vi "test_rw_string.vi"(8 "error in (no error)":errorcluster) -> (0 "error out":errorcluster)   [LabVIEW 2020]
uses:
  75441b51-3bf2-4981-8bbc-1672bc4a7a0b.vi
  75441b51-3bf2-4981-8bbc-1672bc4a7a0b.vi/4178f046-9af6-4db4-9405-99552d650b27.vi
  75441b51-3bf2-4981-8bbc-1672bc4a7a0b.vi/504846f3-46c1-483c-ab2c-e4b1da560c38.vi
  toml/write_subtable_key_string.vi
  toml/toml.lvclass
  <vilib>/addons/_JKI Toolkits/Caraya/classes/Assert/Assert.lvclass
  <vilib>/addons/_JKI Toolkits/Caraya/classes/Test/Test.lvclass
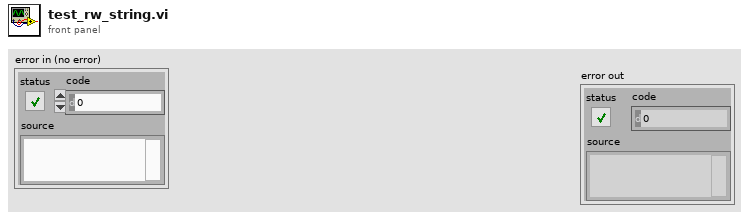
[diagram p1: front panel]
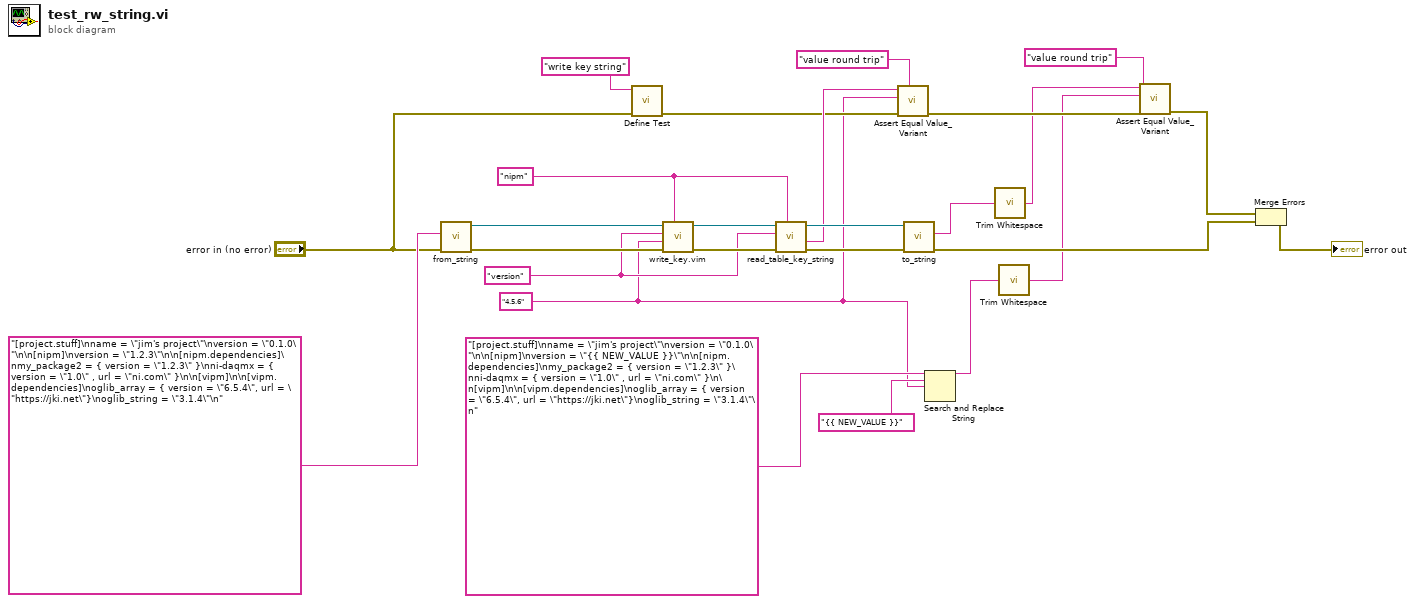
[diagram p0: block diagram]
diagram:
  w2 = "version" ("table_name")
  w3 = "nipm" ("table_name")
  w1 = "4.5.6" ("string")
  n1 = call "from_string.vi"("error in (no error)"="error in (no error)", "toml"="[project.stuff]\nname = \"jim's project\"\nversion = \"0.1.0\"\n\n[nipm]\nversion = \"1.2.3\"\n\n[nipm.dependencies]\nmy_package2 = { version = \"1.2.3\" }\nni-daqmx = { version = \"1.0\" , url = \"ni.com\" }\n\n[vipm]\n\n[vipm.dependencies]\noglib_array = { version = \"6.5.4\", url = \"https://jki.net\"}\noglib_string = \"3.1.4\"\n" ("toml_string in")) -> ("error out"=w21:errorcluster, "toml out"=w20:refnum<class "toml.lvclass">)  [unwired: 8 in]
  n2 = call <vilib>:"Define Test.vi"("error in (no error)"="error in (no error)", "Label (VI Title)"="write key string") -> ("error out"=w9:errorcluster)  [unwired: 9 in]
  n3 = call "write_key.vim"("table"=w3, "error in (no error)"=w21, "value"=w1, "key"=w2, "toml in"=w20) -> ("error out"=w25:errorcluster, "toml out"=w23:refnum<class "toml.lvclass">)  [unwired: 5 in]
  n4 = call "read_table_key_string.vi"("table"=w3, "error in (no error)"=w25, "key"=w2, "toml in"=w23) -> ("error out"=w24:errorcluster, "value"=w19:string, "toml out"=w22:refnum<class "toml.lvclass">)  [unwired: 4 in, 1 out]
  n5 = call <vilib>:"Assert Equal Value_Variant.vi"("Label"="value round trip", "error in (no error)"=w9, "Y"=w1, "X"=w19) -> ("error out"=w18:errorcluster)  [unwired: 7 in]
  n6 = call "to_string.vi"("error in (no error)"=w24, "toml in"=w22) -> ("error out"=w15:errorcluster, "toml_string"=w7:string)  [unwired: 8 in]
  n7 = Search and Replace String(input string="[project.stuff]\nname = \"jim's project\"\nversion = \"0.1.0\"\n\n[nipm]\nversion = \"{{ NEW_VALUE }}\"\n\n[nipm.dependencies]\nmy_package2 = { version = \"1.2.3\" }\nni-daqmx = { version = \"1.0\" , url = \"ni.com\" }\n\n[vipm]\n\n[vipm.dependencies]\noglib_array = { version = \"6.5.4\", url = \"https://jki.net\"}\noglib_string = \"3.1.4\"\n" ("toml_string in"), search string="{{ NEW_VALUE }}", replace string=w1) -> (result string=w5:string)  [unwired: 5 in, 3 out]
  n8 = call <vilib>:"Trim Whitespace.vi"("string"=w7) -> ("trimmed string"=w6:string)  [unwired: 1 in]
  n9 = call <vilib>:"Trim Whitespace.vi"("string"=w5) -> ("trimmed string"=w4:string)  [unwired: 1 in]
  n10 = call <vilib>:"Assert Equal Value_Variant.vi"("Label"="value round trip", "error in (no error)"=w18, "Y"=w4, "X"=w6) -> ("error out"=w16:errorcluster)  [unwired: 7 in]
  n11 = Merge Errors(w16, w15) -> (→"error out":errorcluster)
